vi "West Eq.vi"(4 "O2%":dbl=15.0, 6 "Pressure Pa":dbl=101334.0, 7 "Air pressure Pa":dbl=85234.27 format="%.2f", 8 "Alt M":dbl=1524.0) -> (1 "Alt Eff M 1 correct":dbl, 2 "Alt M":dbl=1510.833483871793, 3 "Pressure 2 correct":dbl=85234.27456503273 format="%.2f")   [LabVIEW 2012]
panel:
  out "Alt Eff M 2 correct":dbl=2725.698552346179
  out "Ratio":dbl=0.7163960050816649
  out "PO2":dbl=15200.1
  out "Alt 2 correct":dbl=1524.3393032524548
  out "Air pressure Pa incorrect":dbl=85826.25079728545
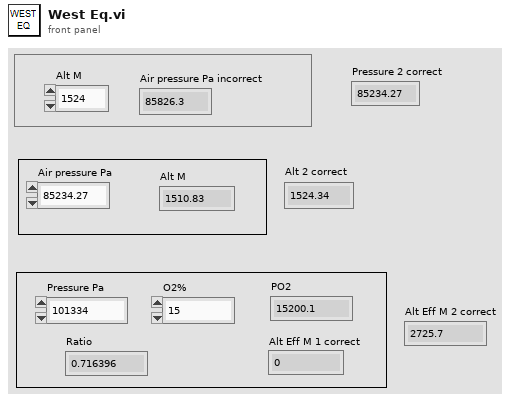
[diagram p1: front panel]
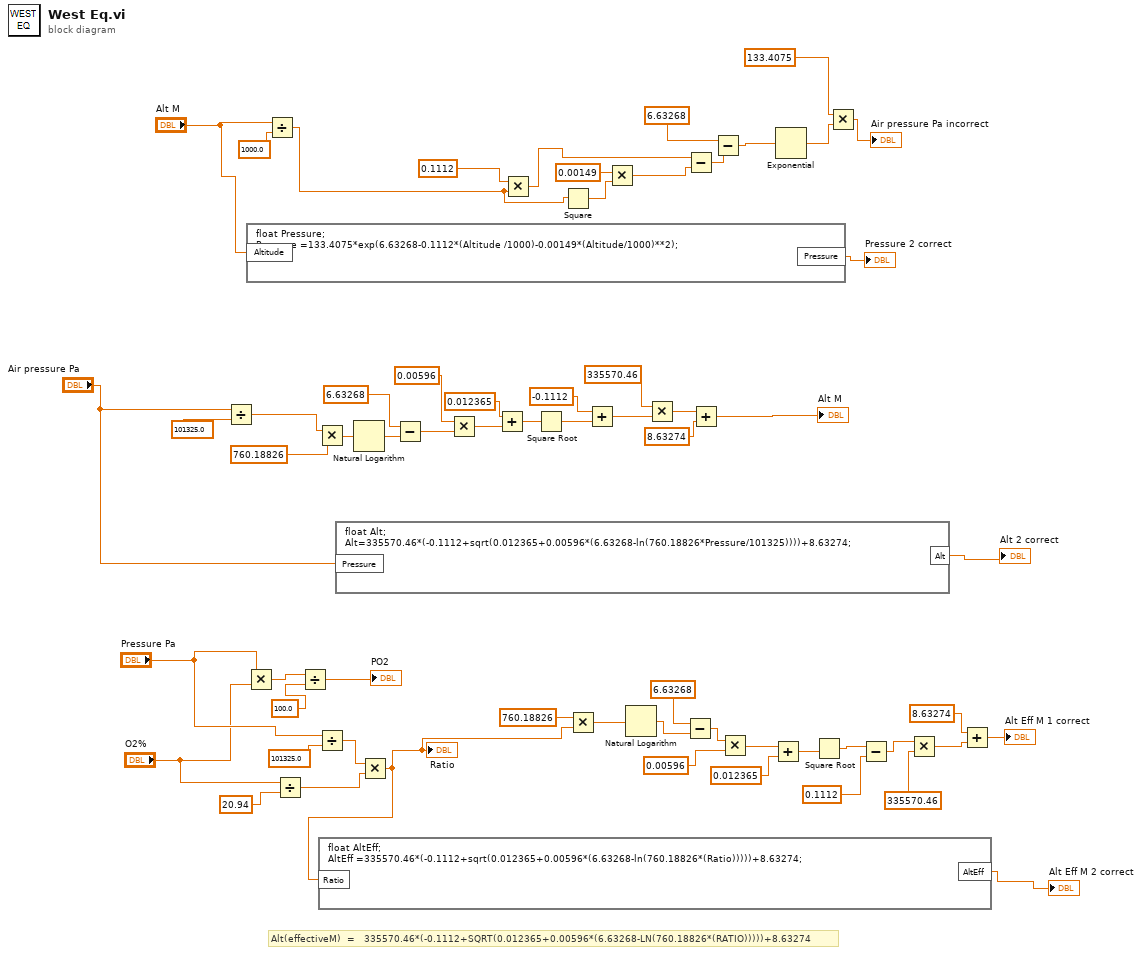
[diagram p0: block diagram]
diagram:
  # "Alt(effectiveM)  =   335570.46*(-0.1112+SQRT(0.012365+0.00596*(6.63268-LN(760.18826*(RATIO)))))+8.63274"
  n1 = Divide(x="Air pressure Pa", y=101325.0) -> (x/y=w52:dbl)
  n2 = Multiply(x="Pressure Pa", y="O2%") -> (x*y=w62:dbl)
  n3 = formula code="float Pressure;\nPressure =133.4075*exp(6.63268-0.1112*(Altitude /1000)-0.00149*(Altitude/1000)**2);"("Altitude"="Alt M") -> ("Pressure"=→"Pressure 2 correct":dbl)
  n4 = Divide(x="Alt M", y=1000.0) -> (x/y=w7:dbl)
  n5 = Divide(x="O2%", y=20.94) -> (x/y=w57:dbl)
  n6 = Divide(x=w62, y=100.0 ("x")) -> (x/y=→"PO2":dbl)
  n7 = Multiply(x=w52, y=760.18826) -> (x*y=w50:dbl)
  n8 = Divide(x="Pressure Pa", y=101325.0) -> (x/y=w56:dbl)
  n9 = formula code="float Alt;\nAlt=335570.46*(-0.1112+sqrt(0.012365+0.00596*(6.63268-ln(760.18826*Pressure/101325))))+8.63274;"("Pressure"="Air pressure Pa") -> ("Alt"=→"Alt 2 correct":dbl)
  n10 = Natural Logarithm(1:w50) -> (0:w42:dbl)
  n11 = Multiply(x=w56, y=w57) -> (x*y=w30:dbl)
  "Ratio" <- w30
  n12 = formula code="float AltEff;\nAltEff =335570.46*(-0.1112+sqrt(0.012365+0.00596*(6.63268-ln(760.18826*(Ratio)))))+8.63274;"("Ratio"=w30) -> ("AltEff"=→"Alt Eff M 2 correct":dbl)
  n13 = Subtract(x=6.63268, y=w42) -> (x-y=w38:dbl)
  n14 = Multiply(x=0.00596, y=w38) -> (x*y=w44:dbl)
  n15 = Add(x=0.012365, y=w44) -> (x+y=w37:dbl)
  n16 = Multiply(x=0.1112, y=w7) -> (x*y=w9:dbl)
  n17 = Square Root(x=w37) -> (sqrt(x)=w48:dbl)
  n18 = Square(x=w7) -> (x^2=w5:dbl)
  n19 = Multiply(x=760.18826, y=w30) -> (x*y=w29:dbl)
  n20 = Add(x=-0.1112, y=w48) -> (x+y=w39:dbl)
  n21 = Multiply(x=0.00149, y=w5) -> (x*y=w4:dbl)
  n22 = Natural Logarithm(1:w29) -> (0:w27:dbl)
  n23 = Multiply(x=335570.46, y=w39) -> (x*y=w46:dbl)
  n24 = Subtract(x=6.63268, y=w27) -> (x-y=w26:dbl)
  n25 = Subtract(x=w9, y=w4) -> (x-y=w8:dbl)
  n26 = Add(x=w46, y=8.63274) -> (x+y=→"Alt M":dbl)
  n27 = Subtract(x=6.63268, y=w8) -> (x-y=w3:dbl)
  n28 = Multiply(x=w26, y=0.00596 ("x")) -> (x*y=w24:dbl)
  n29 = Add(x=w24, y=0.012365 ("x")) -> (x+y=w22:dbl)
  n30 = Exponential(1:w3) -> (0:w2:dbl)
  n31 = Square Root(x=w22) -> (sqrt(x)=w21:dbl)
  n32 = Multiply(x=133.4075, y=w2) -> (x*y=→"Air pressure Pa incorrect":dbl)
  n33 = Subtract(x=w21, y=0.1112 ("x")) -> (x-y=w19:dbl)
  n34 = Multiply(x=w19, y=335570.46 ("x")) -> (x*y=w17:dbl)
  n35 = Add(x=8.63274, y=w17) -> (x+y=→"Alt Eff M 1 correct":dbl)
